vi "Do.vi"(8 "error in (no error)":errorcluster, 9 "Events":refnum<class "Events.lvclass">, 10 "Message Loop Data in":T1, 11 "IUnsubscribe in":refnum<class "IUnsubscribe.lvclass">) -> (0 "error out":errorcluster, 1 "Write request":T9, 2 "Message Loop Data out":T1, 3 "IUnsubscribe out":refnum<class "IUnsubscribe.lvclass">)   [LabVIEW 2020, in "wamplv.lvlib" / "IUnsubscribe.lvclass"]
uses:
  IUnsubscribe.lvclass
  wamplv.lvlib
  WAMP Client/Private/TypeDef/Publish Requests Map.ctl
  WAMP Client/Private/TypeDef/Endpoint Data.ctl
  Call/ICallRequest/ICallRequest.lvclass
  WAMP Client/Private/TypeDef/CALL Request Map.ctl
  WAMP Client/Private/TypeDef/SUBSCRIBE Requests Map.ctl
  WAMP Client/Private/TypeDef/Subscriptions Map.ctl
  WAMP Client/Private/TypeDef/Unsubscribe Requests Map.ctl
  WAMP Client/Private/TypeDef/Unregister requests map.ctl
  WAMP Client/Private/TypeDef/Message Loop Data.ctl
  TypeDefs/Transport type.ctl
  WAMP Client/Private/TypeDef/Write queue item.ctl
  Events/EventsParent/Events.lvclass
  Subscribe/ISubscribe/ISubscribe.lvclass
  Publish/IPublish/IPublish.lvclass
  Message loop classes/Subscription details/SubscriptionDetailsParent/SubscriptionDetailsParent.lvclass
  Register/IRegister/IRegister.lvclass
  Unregister/IUnregister/IUnregister.lvclass
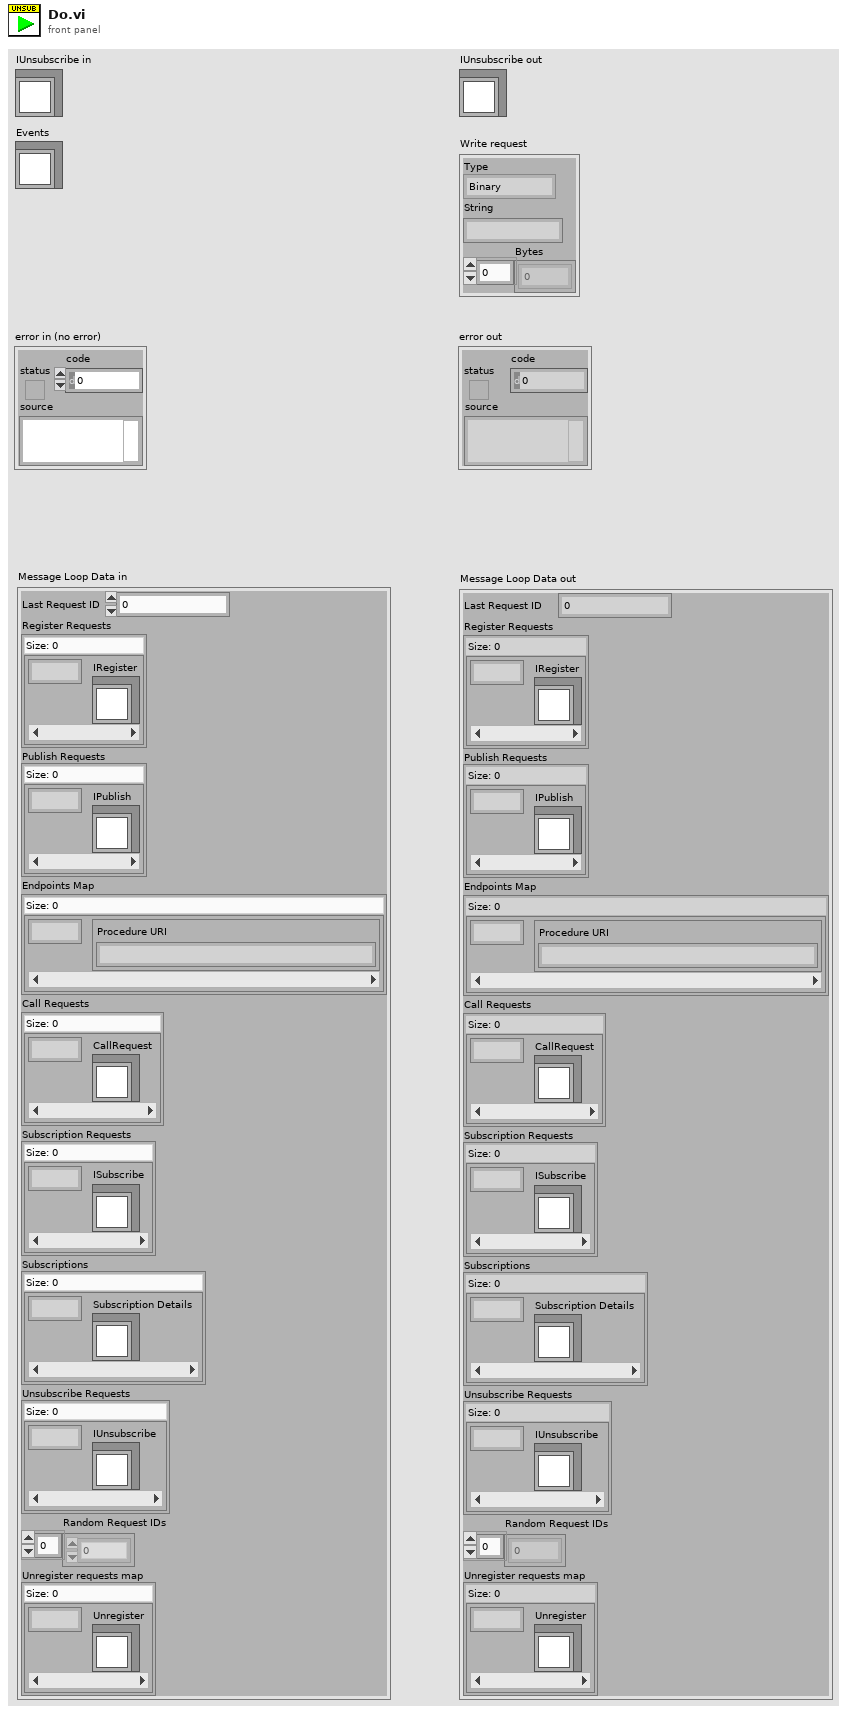
[diagram p1: front panel]
types:
  T1 = typedef "wamplv.lvlib/Message Loop Data.ctl" = cluster{"Last Request ID":u64, "Register Requests":map{u64, refnum<class "IRegister.lvclass">}, "Publish Requests":T2, "Endpoints Map":map{u64, T3}, "Call Requests":T4, "Subscription Requests":T5, "Subscriptions":T6, "Unsubscribe Requests":T7, "Random Request IDs":u64[], "Unregister requests map":T8}
  T2 = typedef "wamplv.lvlib/Publish Requests Map.ctl" = map{u64, refnum<class "IPublish.lvclass">}
  T3 = typedef "wamplv.lvlib/Endpoint Data.ctl" = cluster{"Procedure URI":string}
  T4 = typedef "wamplv.lvlib/CALL Request Map.ctl" = map{u64, refnum<class "ICallRequest.lvclass">}
  T5 = typedef "wamplv.lvlib/SUBSCRIBE Requests Map.ctl" = map{u64, refnum<class "ISubscribe.lvclass">}
  T6 = typedef "wamplv.lvlib/Subscriptions Map.ctl" = map{u64, refnum<class "SubscriptionDetailsParent.lvclass">}
  T7 = typedef "wamplv.lvlib/Unsubscribe Requests Map.ctl" = map{u64, refnum<class "IUnsubscribe.lvclass">}
  T8 = typedef "wamplv.lvlib/Unregister requests map.ctl" = map{u64, refnum<class "IUnregister.lvclass">}
  T9 = typedef "wamplv.lvlib/Write queue item.ctl" = cluster{"Type":T10, "String":string, "Bytes":u8[]}
  T10 = typedef "wamplv.lvlib/Transport type.ctl" = enum16{"Binary", "Text"}
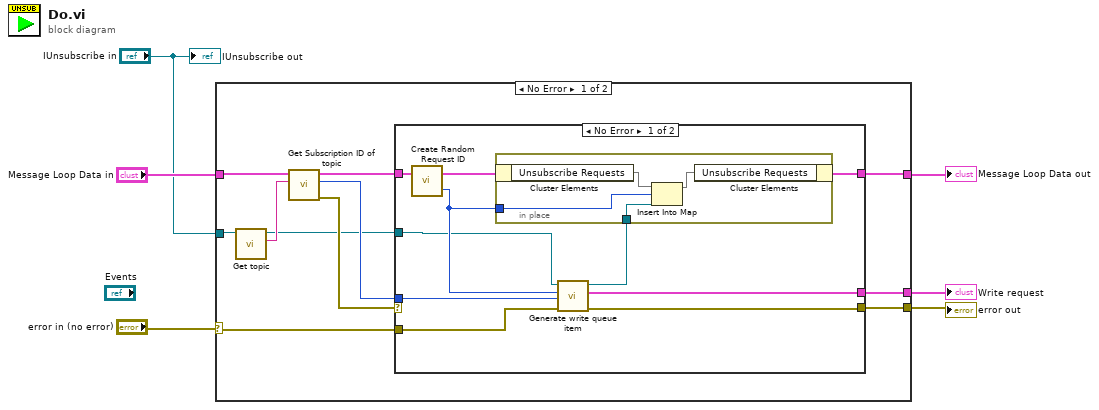
[diagram p0: block diagram]
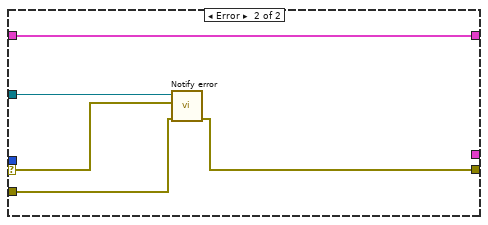
[diagram p2: hidden frame]
diagram:
  n1 = case shown="No Error" "error in (no error)" {
    selector: "error in (no error)" -> [w7 w38]
    tunnel: [w17 w38] -> w3
    tunnel: "IUnsubscribe in" -> [w11 _]
    tunnel: "Message Loop Data in" -> [w14 w37]
    tunnel: [w12 w37] -> w5
    tunnel: [w8 _] -> w1
    frame No Error {
      n2 = call-dynamic "Get topic.vi"("IUnsubscribe in"=w11) -> ("Topic URl"=w10:string, "IUnsubscribe out"=w9:refnum<class "IUnsubscribe.lvclass">)  [unwired: 9 in]
      n3 = call "Get Subscription ID of topic.vi"("Topic"=w10, "Message loop data (in)"=w14) -> ("error out"=w13:errorcluster, "Subscription ID"=w16:u64, "Message loop data (out)"=w15:T1)  [unwired: 7 in]
      n4 = case shown="No Error" w13 {
        selector: w13 -> [_ w34]
        tunnel: [w20 w33] -> w17
        tunnel: w16 -> [w23 _]
        tunnel: w9 -> [w21 w35]
        tunnel: w15 -> [w27 w36]
        tunnel: [w25 w36] -> w12
        tunnel: [w19 _] -> w8
        tunnel: w7 -> [w18 w32]
        frame No Error {
          n5 = call "Create Random Request ID.vi"("Message Loop Shift Register Data (in)"=w27) -> ("Generated Request ID"=w24:u64, "Message Loop Shift Register Data (out)"=w26:T1)  [unwired: 1 in]
          n6 = call-dynamic "Generate write queue item.vi"("error in (no error)"=w18, "Subscription ID"=w23, "Request ID"=w24, "IUnsubscribe in"=w21) -> ("error out"=w20:errorcluster, "Write queue item"=w19:T9, "IUnsubscribe out"=w22:refnum<class "IUnsubscribe.lvclass">)  [unwired: 5 in]
          n7 = in-place "In Place Element Structure" {
            in-place-border: w24 -> [w31]
            in-place-border: w22 -> [w30]
            n8 = in-place-cluster #1(w26) -> ("Unsubscribe Requests"=w29:T7)
            n9 = Insert Into Map(map in=w29, key=w31, value=w30) -> (map out=w28:T7)  [unwired: 2 out]
            n10 = in-place-cluster #1("Unsubscribe Requests"=w28) -> (w25:T1)
          }
        }
        frame Error {
          n11 = call-dynamic "Notify error.vi"("error in (no error)"=w32, "Unsubscribe error"=w34, "IUnsubscribe in"=w35) -> ("error out"=w33:errorcluster)  [unwired: 7 in, 1 out]
        }
      }
    }
    frame Error {
    }
  }
  "error out" <- w3
  "Write request" <- w1
  "Message Loop Data out" <- w5
  "IUnsubscribe out" <- "IUnsubscribe in"
